vi "Pump Concentrations in Procent.vi"(11 "Pump Concetrations-Cluster (Eingang)":T1) -> (3 "Pump Concetrations-Cluster (Ausgang)":T1)   [LabVIEW 2020, in "Linearisierung v2.lvlib" / "Gasteiler.lvlib" / "HovaCAL_Interface.lvlib" / "Helper.lvlib"]
uses:
  Helper.lvlib
  Controls/Pump Concentration.ctl
  Controls/Controls.lvlib
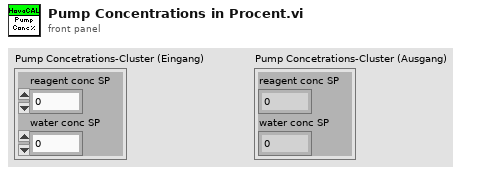
[diagram p1: front panel]
types:
  T1 = typedef "Linearisierung v2.lvlib/Gasteiler.lvlib/HovaCAL_Interface.lvlib/Controls.lvlib/Pump Concentration.ctl" = cluster{"reagent conc SP":dbl, "water conc SP":dbl}
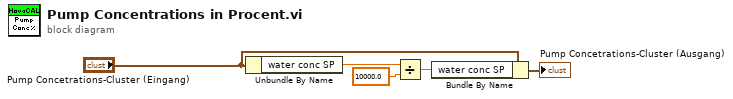
[diagram p0: block diagram]
diagram:
  n1 = Unbundle By Name("Pump Concetrations-Cluster (Eingang)") -> ("water conc SP"=w4:dbl)
  n2 = Divide(x=w4, y=10000.0) -> (x/y=w3:dbl)
  n3 = Bundle By Name(cluster="Pump Concetrations-Cluster (Eingang)", "water conc SP"=w3) -> (→"Pump Concetrations-Cluster (Ausgang)":T1)
